vi "PH_IEEE1394Camera.evt call SetBrightness.vi"(0 "i ref in":refnum<vi>, 2 "Instance":string, 3 "Brightness":dbl, 5 "error in (no error)":errorcluster) -> (14 "i ref out":refnum<vi>, 19 "error out":errorcluster)   [LabVIEW 2014, in "PH_IEEE1394Camera.lvlib"]
doc: "This VI sends a simple call for SetBrightness."
uses:
  PH_IEEE1394Camera.lvlib
  CS_Core/CSSystem/CoreLib/CoreLib.double 2 byte array.vi
  CS_Core/CSSystem/CoreLib/CoreLib.lvlib
  CS_Core/BaseProcess/BaseProcess.lvlib
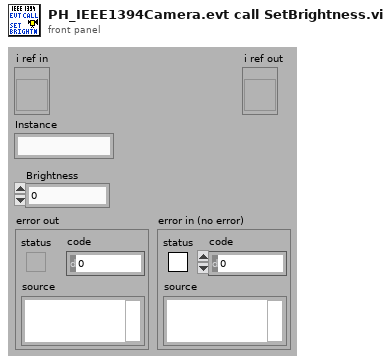
[diagram p1: front panel]
types:
  T1 = typedef "CoreDefs.rawDataType.ctl" = i8[]
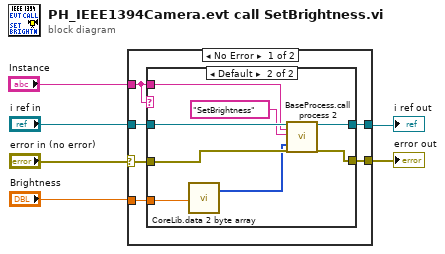
[diagram p0: block diagram]
diagram:
  n1 = case shown="No Error" "error in (no error)" {
    selector: "error in (no error)" -> [w9 w23]
    tunnel: [w12 w24] -> w4
    tunnel: [w11 w23] -> w3
    tunnel: "i ref in" -> [w10 w24]
    tunnel: "Instance" -> [w8 _]
    tunnel: "Brightness" -> [w7 _]
    frame No Error {
      n2 = case shown="Default" w8 {
        tunnel: [w14 w22] -> w12
        tunnel: [w13 w21] -> w11
        tunnel: w10 -> [w14 w20]
        tunnel: w8 -> [_ w19]
        tunnel: w9 -> [w13 w17]
        tunnel: w7 -> [_ w15]
        frame "N/A" {
        }
        frame Default {
          n3 = call-poly "CoreLib.data 2 byte array.vi"("f64"=w15) -> ("byteArray out"=w16:T1)  [unwired: 18 in]
          n4 = call "BaseProcess.call process 2.vi"("i ref in"=w20, "Object"=w19, "Selector"="SetBrightness", "Data"=w16, "error in (no error)"=w17) -> ("i ref out"=w22:refnum<vi>, "error out"=w21:errorcluster)  [unwired: 13 in]
        }
      }
    }
    frame Error {
    }
  }
  "error out" <- w3
  "i ref out" <- w4
